vi "Global_HW Status.vi"() -> ()   [LabVIEW 2017, in "Hopper System.lvlib"]
uses:
  Hopper System.lvlib
panel:
  in  "Balls Shot_HW":i32
  out "Hopper Line BallShot_HW":bool
  out "Hopper Line BallPresent_HW":bool
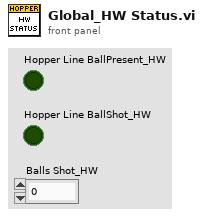
[diagram p1: front panel]
diagram:
